vi "Read from Hardware.vi"(8 "error in":errorcluster, 10 "Values in":dbl[](array[numeric]), 11 "Ballard ARINC-429 Rx Execution Unit in":refnum<class "Ballard ARINC-429 Rx Execution Unit.lvclass">) -> (0 "error out":errorcluster, 2 "Values out":dbl[](array[numeric]), 3 "Ballard ARINC-429 Rx Execution Unit out":refnum<class "Ballard ARINC-429 Rx Execution Unit.lvclass">)   [LabVIEW 2020, in "Ballard ARINC 429 Engine.lvlib" / "Implementation.lvlib" / "Ballard ARINC-429 Rx Execution Unit.lvclass"]
uses:
  Ballard ARINC-429 Rx Execution Unit.lvclass
  C:/Git/niveristand-ballard-arinc429-custom-device/Source/Custom Device Support/Engine/Implementation/Ballard ARINC-429 Execution Unit/Ballard ARINC-429 Execution Unit.lvclass
  Ballard ARINC-429 Execution Unit/Ballard ARINC-429 Execution Unit.lvclass/Ballard ARINC-429 Execution Unit.ctl
  Ballard ARINC-429 Rx Execution Unit.lvclass/Ballard ARINC-429 Rx Execution Unit.ctl
  Read Map.vi
  Read RT hardware channels.vi
  Read Status Error Channel Data References.vi
  Ballard ARINC-429 Execution Unit/Ballard ARINC-429 Execution Unit.lvclass
  Custom Device/Custom Device.lvlib
  <instrlib>/BTICardLib/BTICardLV.lvlib
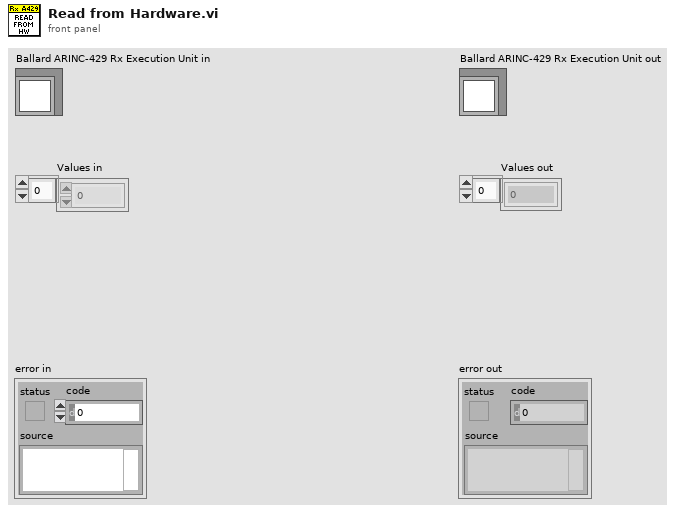
[diagram p1: front panel]
types:
  T1 = typedef "Ballard ARINC 429 Engine.lvlib/Custom Device.lvlib/Hardware Handles.ctl" = cluster{"core handle":u64, "core reader handle":u64, "channel handles":u64[]}
  T2 = cluster{"gap":i16, "parity":i16, "long word":i16, "bit timing":i16, "timeout":i16}
  T3 = map{cluster{"hardware channel":u8, "label":u8, "SDI":u8}, cluster{"data word":u32, "time stamp":dbl}}
  T4 = typedef "BTICardLV.lvlib/429 Record.ctl" = cluster{"type":u16, "count":u16, "timestamp":u32, "msgact":u16, "decgap":u16, "data":u32, "timestamph":u32}
  T5 = cluster{"gap":bool, "parity":bool, "long word":bool, "bit timing":bool, "timeout":bool}
  T6 = cluster{"hardware channel":u8, "label":u8, "SDI":u8}
  T7 = typedef "Map of Identifiers to Indexes.ctl" = map{cluster{"Port":u8, "Label":u8, "SDI":u8}, cluster{"channel index":i32, "label index":i32, "start index":i32, "parameters":i32, "timestamp index":i32}}
  T8 = typedef "RT Hardware Channel Settings.ctl" = cluster{"channel #":u16, "channel handle":u64, "labels settings for RT":T9[]}
  T9 = typedef "RT Label Settings.ctl" = cluster{"Name":string, "xmlName":string, "label":T10, "transfer period":u32, "SDI_Enabled":bool, "SDI":u8, "parameter driver data":T11, "transfer type":T17, "has timestamp?":bool, "Label Disable/Trigger Channel Reference":T16, "Message Handle":u64, "Initialized?":bool, "Word Initial Raw Value":u32, "Label Timestamp Channel Data Reference":T15}
  T10 = typedef "Label.ctl" = u8
  T11 = typedef "RT Parameters.ctl" = cluster{"parameter definitions":T12[], "Rx block data refs":T14[], "Rx values":dbl[], "Tx parameter refs":T16[]}
  T12 = typedef "Parameter Definition.ctl" = cluster{"start index":i32, "size":i32, "encoding":T13, "signed":bool, "scale multiplier":dbl, "scale offset":dbl}
  T13 = typedef "Encoding and Decoding.lvlib/Encoding.ctl" = enum16{"BNR", "BCD", "Discrete"}
  T14 = typedef "Custom Device API.lvlib/Block Data Reference.ctl" = cluster{"Data Reference":T15, "Offset":u64, "Length":u64}
  T15 = typedef "Custom Device API.lvlib/Data Reference.ctl" = i32
  T16 = typedef "Custom Device API.lvlib/Custom Device Item Ref.ctl" = u64
  T17 = typedef "Transfer Type.ctl" = enum16{"Scheduled", "Acyclic", "Block", "Strobe"}
  T18 = cluster{"receiving":T15, "specific errors":cluster{"gap":T15, "parity":T15, "long word ":T15, "bit timing":T15, "timeout":T15}}
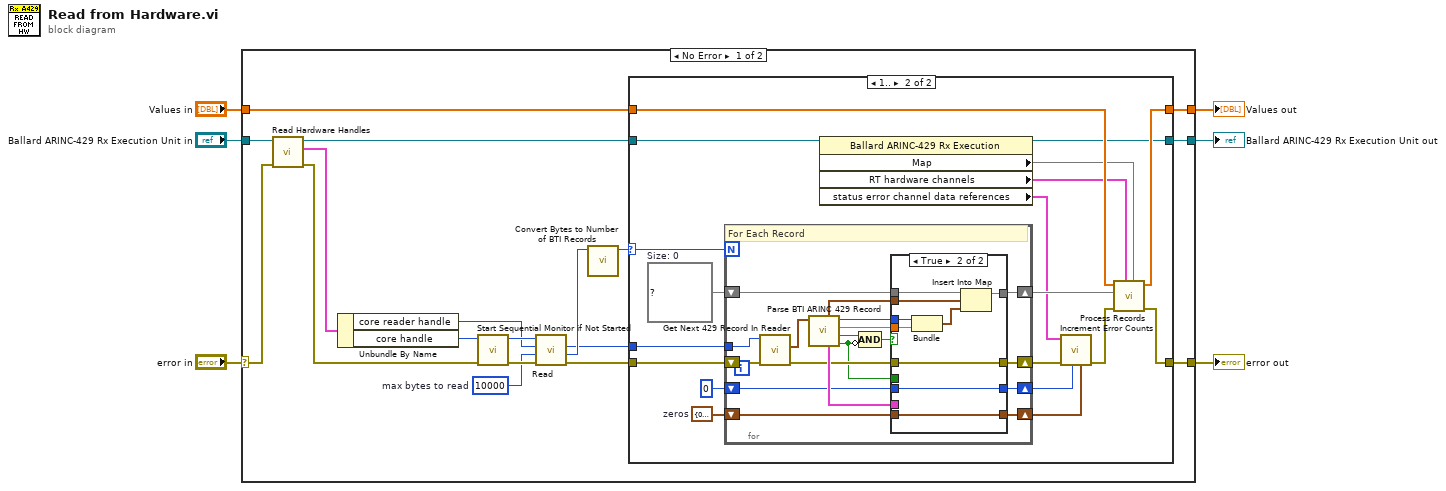
[diagram p0: block diagram]
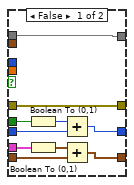
[diagram p3: hidden frame]
diagram:
  n1 = case shown="No Error" "error in" {
    selector: "error in" -> [w24 w85]
    tunnel: [w10 w86] -> w5
    tunnel: "Ballard ARINC-429 Rx Execution Unit in" -> [w23 w86]
    tunnel: [w9 w85] -> w3
    tunnel: [w8 w84] -> w2
    tunnel: "Values in" -> [w7 w84]
    frame No Error {
      w16 = 10000  # max bytes to read
      n2 = call "Read Hardware Handles.vi"("error in"=w24, "Ballard ARINC-429 Execution Unit in"=w23) -> ("error out"=w20:errorcluster, "hardware handles"=w22:T1, "Ballard ARINC-429 Execution Unit out"=w11:refnum<class "Ballard ARINC-429 Rx Execution Unit.lvclass">)  [unwired: 7 in]
      n3 = Unbundle By Name(w22) -> ("core reader handle"=w18:u64, "core handle"=w21:u64)
      n4 = call "Start Sequential Monitor if Not Started.vi"("error in"=w20, "core handle in"=w21) -> ("error out"=w17:errorcluster, "core handle out"=w19:u64)  [unwired: 8 in]
      n5 = call <instrlib>:"Read.vi"("error in (no error)"=w17, "max bytes to read"=w16, "core reader handle in"=w18, "core handle in"=w19) -> ("error out"=w12:errorcluster, "bytes read"=w15:i32, "core reader handle out"=w13:u64)  [unwired: 4 in, 1 out]
      n6 = call "Convert Bytes to Number of BTI Records.vi"("bytes read"=w15) -> ("number of records read"=w14:i32)  [unwired: 10 in]
      n7 = case shown="1.." w14 {
        selector: w14 -> [_ w46]
        tunnel: w13 -> [_ w45]
        tunnel: w12 -> [w26 w44]
        tunnel: w11 -> [w27 w40]
        tunnel: [w27 w39] -> w10
        tunnel: [w26 w43] -> w9
        tunnel: [w25 w42] -> w8
        tunnel: w7 -> [w25 w41]
        frame Default {
        }
        frame 1.. {
          w34 = T2 {"gap"=0, "parity"=0, "long word"=0, "bit timing"=0, "timeout"=0}  # zeros
          w36 = T3 {}  # Size: 0
          n8 = for {
            N: w46 -> [_]
            tunnel: w45 -> [w64]
            shift-right: [w50] -> w32
            shift-left: w44 -> [w63]
            shift-right: [w58] -> w35
            shift-left: w36 -> [w57]
            shift-right: [w56] -> w28
            shift-left: w34 -> [w55]
            shift-right: [w48] -> w29
            shift-left: i16 0 -> [w47]
            # "For Each Record"
            n9 = call <instrlib>:"Get Next 429 Record In Reader.vi"("error in (no error)"=w63, "core reader handle in"=w64) -> ("error out"=w51:errorcluster, "record out"=w62:T4)  [unwired: 7 in, 1 out]
            n10 = call "Parse BTI ARINC 429 Record.vi"("record"=w62) -> ("receiving error"=w49:bool, "hit"=w53:bool, "time stamp"=w61:dbl, "data word"=w60:u32, "specific errors"=w54:T5, "message info"=w59:T6)  [unwired: 5 in]
            n11 = Compound Arithmetic op=AND(w53, invert w49) -> (w52:bool)
            n12 = case shown="True" w52 {
              tunnel: w60 -> [_ w80]
              tunnel: w59 -> [_ w81]
              tunnel: [w74 w83] -> w58
              tunnel: w57 -> [w74 w82]
              tunnel: w55 -> [w72 w78]
              tunnel: [w68 w78] -> w56
              tunnel: w61 -> [_ w77]
              tunnel: w54 -> [w71 _]
              tunnel: w51 -> [w70 w76]
              tunnel: [w70 w76] -> w50
              tunnel: w49 -> [w69 _]
              tunnel: [w67 w75] -> w48
              tunnel: w47 -> [w65 w75]
              frame False {
                n13 = Boolean To (0,1)(Boolean=w69) -> (0, 1=w66:i16)
                n14 = Boolean To (0,1)(Boolean=w71) -> (0, 1=w73:T2)
                n15 = Add(x=w66, y=w65) -> (x+y=w67:i16)
                n16 = Add(x=w73, y=w72) -> (x+y=w68:T2)
              }
              frame True {
                n17 = Bundle("data word"=w80, "time stamp"=w77) -> (w79:cluster{"data word":u32, "time stamp":dbl})  [unwired: 1 in]
                n18 = Insert Into Map(map in=w82, key=w81, value=w79) -> (map out=w83:T3)  [unwired: 2 out]
              }
            }
          }
          n19 = property class="Ballard ARINC-429 Rx Execution "(reference=w40) -> (reference out=w39:refnum<class "Ballard ARINC-429 Rx Execution Unit.lvclass">, "Map"=w38:T7, "RT hardware channels"=w37:T8[], "status error channel data references"=w30:T18)  [unwired: 1 in, 1 out]
          n20 = call "Increment Error Counts.vi"("specific errors"=w28, "receiving errors"=w29, "error in"=w32, "status error channel data references"=w30) -> ("error out"=w31:errorcluster)  [unwired: 7 in]
          n21 = call "Process Records.vi"("map from message info to indexes"=w38, "RT hardware channel data"=w37, "error in"=w31, "map from message info to data word"=w35, "parameter values in"=w41) -> ("error out"=w43:errorcluster, "parameter values out"=w42:dbl[])  [unwired: 3 in]
        }
      }
    }
    frame Error {
    }
  }
  "error out" <- w3
  "Ballard ARINC-429 Rx Execution Unit out" <- w5
  "Values out" <- w2
